vi "Module Cleanup.vi"(8 "error in (no error)":errorcluster, 11 "Git Updater Module in":refnum<class "Git Updater Module.lvclass">) -> (0 "error out":errorcluster, 3 "Git Updater Module out":refnum<class "Git Updater Module.lvclass">)   [LabVIEW 2020, in "VolatusGUI.lvlib" / "Git Updater Module.lvclass"]
uses:
  Git Updater Module.lvclass
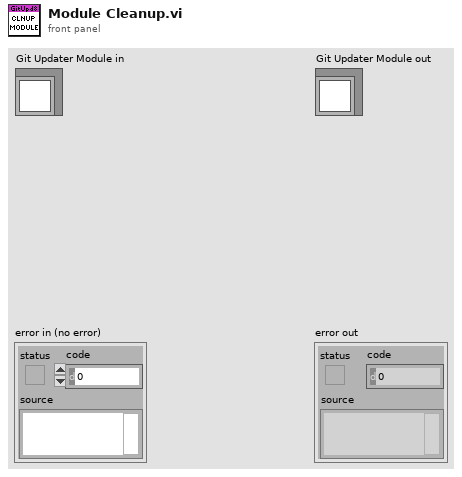
[diagram p1: front panel]
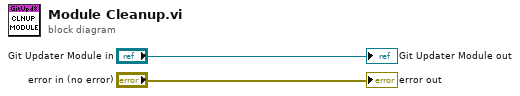
[diagram p0: block diagram]
diagram:
  "error out" <- "error in (no error)"
  "Git Updater Module out" <- "Git Updater Module in"
